vi "Open Listening Server Reference.vi"(8 "error in (no error)":errorcluster, 11 "Plugin in":refnum<class "Generic Plugin.lvclass">) -> (0 "error out":errorcluster, 2 "vi reference":refnum<vi>, 3 "Plugin out":refnum<class "Generic Plugin.lvclass">)   [LabVIEW 2020, in "RxnRover.lvlib" / "Generic Plugin.lvclass"]
uses:
  Generic Plugin.lvclass
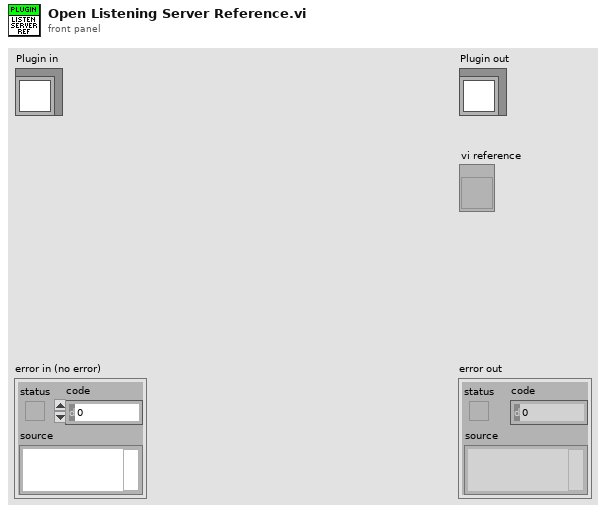
[diagram p1: front panel]
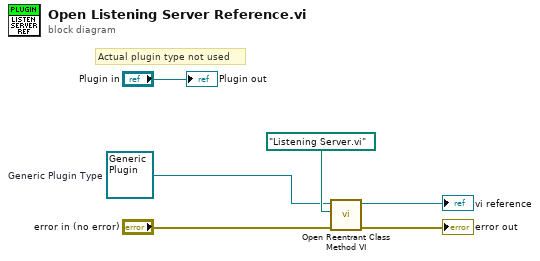
[diagram p0: block diagram]
diagram:
  w1 = refnum<class "Generic Plugin.lvclass"> refnum  # Generic Plugin Type
  # "Actual plugin type not used"
  n1 = call "Open Reentrant Class Method VI.vi"("error in (no error)"="error in (no error)", "Method VI Filename to Open"=path "Listening Server.vi" ("name or relative path"), "Generic Plugin in"=w1) -> ("error out"=→"error out":errorcluster, "VI Refnum"=→"vi reference":refnum<vi>)  [unwired: 7 in]
  "Plugin out" <- "Plugin in"
